vi "Get Object Dependencies.vi"(8 "error in (no error)":errorcluster, 11 "Object":variant) -> (0 "error out":errorcluster, 2 "values":variant[](array[variant]), 3 "Variant":variant)   [LabVIEW 2019, in "JSON-Schema.lvlib"]
uses:
  JSON-Schema.lvlib
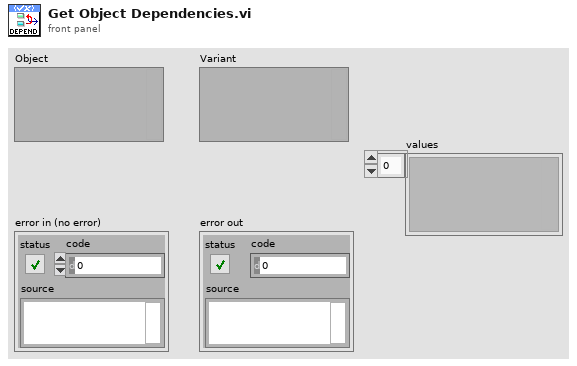
[diagram p1: front panel]
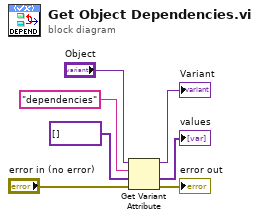
[diagram p0: block diagram]
diagram:
  n1 = Get Variant Attribute(Variant="Object", name="dependencies", default value (empty Variant)=variant[] [], error in="error in (no error)") -> (duplicate Variant=→"Variant":variant, value=→"values":variant[], error out=→"error out":errorcluster)  [unwired: 1 out]
